vi "Read Last run start.vi"(8 "error in (no error)":errorcluster, 11 "Monkey in":refnum<class "Monkey.lvclass">) -> (0 "error out":errorcluster, 2 "Last run start":timestamp, 3 "Monkey out":refnum<class "Monkey.lvclass">)   [LabVIEW 2020, in "TALOS.lvlib" / "Monkey.lvlib" / "Monkey.lvclass"]
uses:
  Monkey.lvclass
  Monkey.lvclass/Monkey.ctl
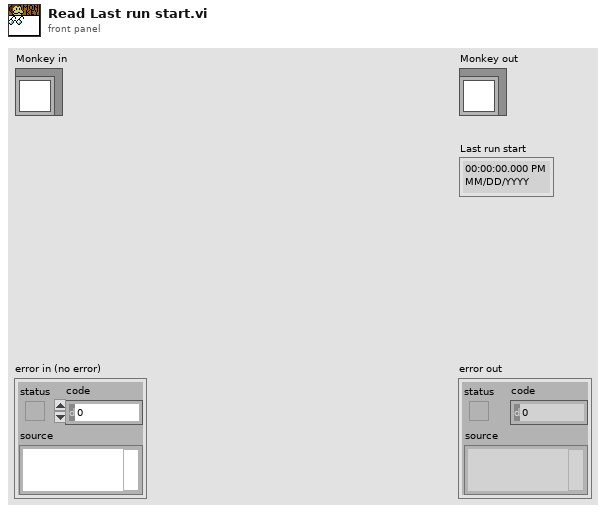
[diagram p1: front panel]
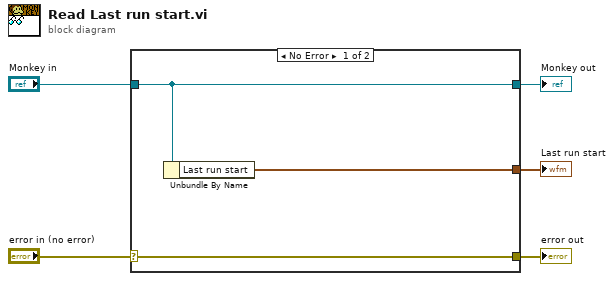
[diagram p0: block diagram]
diagram:
  n1 = case shown="No Error" "error in (no error)" {
    selector: "error in (no error)" -> [w8 w9]
    tunnel: [w8 w9] -> w4
    tunnel: [w7 w10] -> w2
    tunnel: "Monkey in" -> [w7 w10]
    tunnel: [w6 _] -> w1
    frame No Error {
      n2 = Unbundle By Name(w7) -> ("Last run start"=w6:timestamp)
    }
    frame Error {
    }
  }
  "error out" <- w4
  "Monkey out" <- w2
  "Last run start" <- w1
